vi "Format to Technique Parameters.vi"(8 "error in (no error)":errorcluster, 9 "Index":i32, 10 "Internal Technique Parameter":variant, 11 "Potentiostat Galvanostat in":refnum<class "Potentiostat Galvanostat.lvclass">) -> (0 "error out":errorcluster, 2 "Technique Parameters":T1[](array[typedef]) {"Parameter Type" items=["I32 (Long)", "BOOL (Boolean)", "SGL (Single Precision)"]}, 3 "Potentiostat Galvanostat out":refnum<class "Potentiostat Galvanostat.lvclass">)   [LabVIEW 2018, in "Potentiostat Galvanostat.lvclass"]
uses:
  Potentiostat Galvanostat.lvclass
  Controls/Technique Parameter.ctl
  Controls/Parameter Type.ctl
  Controls/Error Codes.ctl
  Potentiostat Galvanostat.lvclass/Potentiostat Galvanostat.ctl
  BL_GetErrorMsg.vi
  <vilib>/Utility/error.llb/Error Cluster From Error Code.vi
  <vilib>/Utility/Data Type/NI_Data Type.lvlib
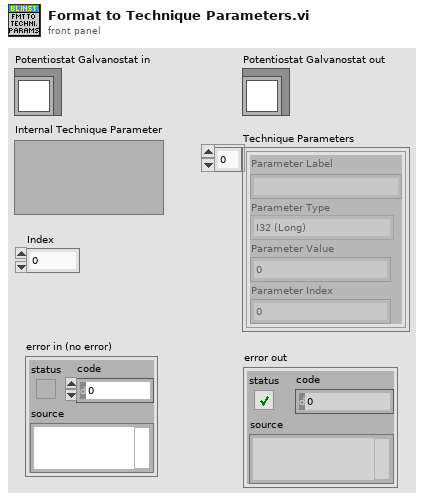
[diagram p1: front panel]
types:
  T1 = typedef "Potentiostat Galvanostat.lvclass/Technique Parameter.ctl" = cluster{"Parameter Label":string, "Parameter Type":T2, "Parameter Value":i32, "Parameter Index":i32}
  T2 = typedef "Potentiostat Galvanostat.lvclass/Parameter Type.ctl" = i32
  T3 = typedef "NI_Data Type.lvlib/Data Type.ctl" = enum8{"Invalid Type", "Void", "I8", "I16", "I32", "I64", "U8", "U16", "U32", "U64", "Single Float", "Double Float", "Extended Float", "Single Complex", "Double Complex", "Extended Complex", "Enum U8", "Enum U16", "Enum U32", "Enum U64", "Single Float With Unit", "Double Float With Unit", "Extended Float With Unit", "Single Complex with Unit", "Double Complex with Unit", "Extended Complex with Unit", "Boolean", "String", "Path", "Picture", "Tag", "Array", "Cluster", "Variant", "LV Variant", "Waveform", "Timestamp", "Digital Waveform", "Digital Data", "ExpressData", "Refnum", "External Data", "VI", "Poly VI", "LabVIEW Class Instance", "Fixed Point"}
  T4 = typedef "Potentiostat Galvanostat.lvclass/Error Codes.ctl" = i32
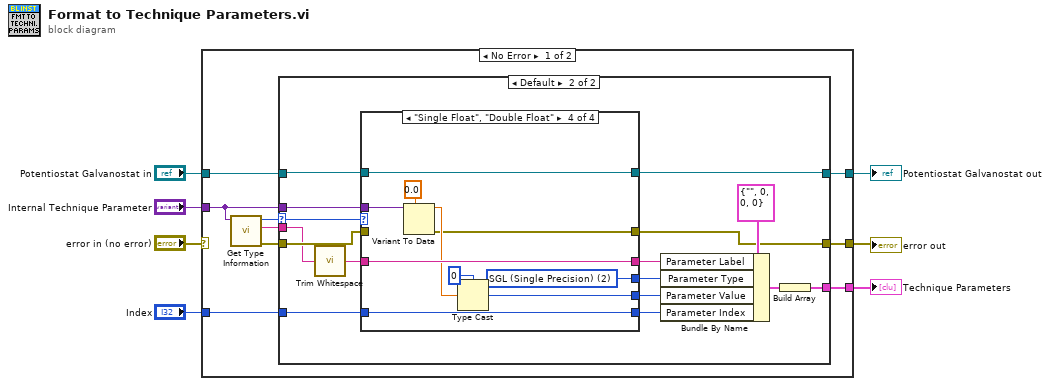
[diagram p0: block diagram]
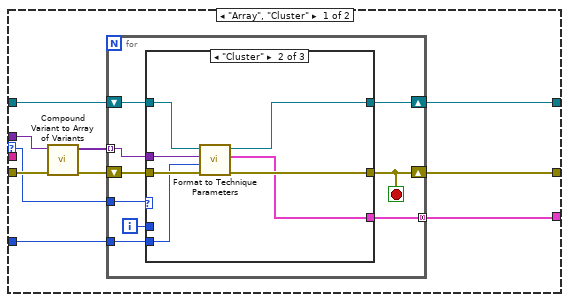
[diagram p2: hidden frame]
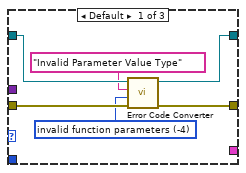
[diagram p3: hidden frame]
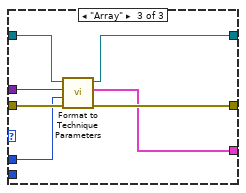
[diagram p4: hidden frame]
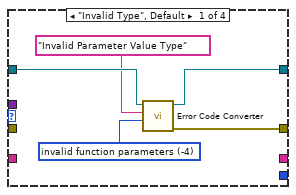
[diagram p5: hidden frame]
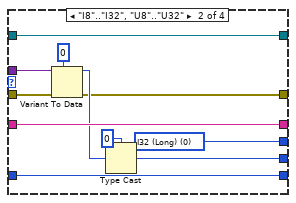
[diagram p6: hidden frame]
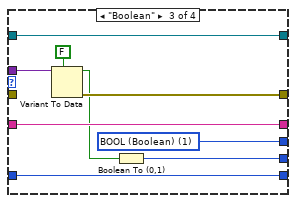
[diagram p7: hidden frame]
diagram:
  n1 = case shown="No Error" "error in (no error)" {
    selector: "error in (no error)" -> [_ w107]
    tunnel: "Internal Technique Parameter" -> [w15 _]
    tunnel: "Index" -> [w12 _]
    tunnel: "Potentiostat Galvanostat in" -> [w11 w108]
    tunnel: [w10 _] -> w4
    tunnel: [w9 w108] -> w3
    tunnel: [w8 w107] -> w2
    frame No Error {
      n2 = call <vilib>:"Get Type Information.vi"("Variant"=w15) -> ("error out"=w13:errorcluster, "Name"=w14:string, "Type"=w16:T3)  [unwired: 6 in, 2 out]
      n3 = case shown="Default" w16 {
        selector: w16 -> [w23 w62]
        tunnel: w15 -> [w26 w64]
        tunnel: w14 -> [_ w61]
        tunnel: w13 -> [w25 w63]
        tunnel: w12 -> [w20 w60]
        tunnel: w11 -> [w22 w65]
        tunnel: [w17 w59] -> w9
        tunnel: [w18 w56] -> w10
        tunnel: [w19 w58] -> w8
        frame "Array", "Cluster" {
          n4 = call "Compound Variant to Array of Variants.vi"("error in (no error)"=w25, "Array/Cluster Variant"=w26) -> ("error out"=w21:errorcluster, "[Variant]"=w24:variant[])  [unwired: 8 in]
          n5 = for {
            tunnel: w24 -> [w33] mode=indexing
            tunnel: w23 -> [w32]
            shift-right: [w29] -> w17
            shift-left: w22 -> [w34]
            shift-right: [w28] -> w19
            shift-left: w21 -> [w35]
            tunnel: w20 -> [w31]
            tunnel: [w30] -> w18 mode=concatenating
            i -> [w27]
            stop <- w28 stop-if-true
            n6 = case shown="\"Cluster\"" w32 {
              tunnel: w35 -> [w38 w48 w55]
              tunnel: w34 -> [w41 w47 w54]
              tunnel: w33 -> [_ w46 w53]
              tunnel: [w37 w45 w52] -> w28
              tunnel: w31 -> [_ w44 _]
              tunnel: [_ w43 w51] -> w30
              tunnel: [w39 w42 w50] -> w29
              tunnel: w27 -> [_ _ w49]
              frame Default {
                w36 = T4 -4 items=["No Error"=0, "no instrument connected"=-1, "connection in progress"=-2, "selected channel(s) unplugged"=-3, "invalid function parameters"=-4, "selected file does not exist"=-5, "function failed"=-6, "no channel selected"=-7, "invalid instrument configuration"=-8, "EC-Lab firmware loaded on the instrument"=-9, "library not correctly loaded in memory"=-10, "USB library not correctly loaded in memory"=-11, "function of the library already in progress"=-12, "selected channel(s) already used"=-13, "device not allowed"=-14, "Invalid update function parameters"=-15, "internal instrument communication failed"=-101, "too many data to transfer from the instrument (device error)"=-102, "selected channel(s) unplugged (device error)"=-103, "instrument response error"=-104, "invalid message size"=-105] ("Error Code")
                n7 = call "Error Code Converter.vi"("error in (no error)"=w38, "Error Code"=w36, "Additional Description"="Invalid Parameter Value Type", "Potentiostat Galvanostat in"=w41) -> ("error out"=w37:errorcluster, "Potentiostat Galvanostat out"=w39:refnum<class "Potentiostat Galvanostat.lvclass">)  [unwired: 6 in]
              }
              frame "Cluster" {
                n8 = call "Format to Technique Parameters.vi"("error in (no error)"=w48, "Index"=w44, "Internal Technique Parameter"=w46, "Potentiostat Galvanostat in"=w47) -> ("error out"=w45:errorcluster, "Technique Parameters"=w43:T1[], "Potentiostat Galvanostat out"=w42:refnum<class "Potentiostat Galvanostat.lvclass">)  [unwired: 5 in]
              }
              frame "Array" {
                n9 = call "Format to Technique Parameters.vi"("error in (no error)"=w55, "Index"=w49, "Internal Technique Parameter"=w53, "Potentiostat Galvanostat in"=w54) -> ("error out"=w52:errorcluster, "Technique Parameters"=w51:T1[], "Potentiostat Galvanostat out"=w50:refnum<class "Potentiostat Galvanostat.lvclass">)  [unwired: 5 in]
              }
            }
          }
        }
        frame Default {
          n10 = call <vilib>:"Trim Whitespace.vi"("string"=w61) -> ("trimmed string"=w71:string)  [unwired: 1 in]
          n11 = case shown="\"Single Float\", \"Double Float\"" w62 {
            tunnel: w64 -> [_ w87 w96 w106]
            tunnel: w65 -> [w76 w78 w90 w97]
            tunnel: [w75 w78 w90 w97] -> w59
            tunnel: [w74 w79 w91 w98] -> w58
            tunnel: w71 -> [_ w85 w94 w104]
            tunnel: w60 -> [_ w84 w93 w103]
            tunnel: [_ w85 w94 w104] -> w67
            tunnel: [_ w80 w92 w99] -> w68
            tunnel: [_ w83 w89 w102] -> w69
            tunnel: [_ w84 w93 w103] -> w70
            tunnel: w63 -> [_ w77 _ _]
            frame "Invalid Type", Default {
              w72 = T4 -4 items=["No Error"=0, "no instrument connected"=-1, "connection in progress"=-2, "selected channel(s) unplugged"=-3, "invalid function parameters"=-4, "selected file does not exist"=-5, "function failed"=-6, "no channel selected"=-7, "invalid instrument configuration"=-8, "EC-Lab firmware loaded on the instrument"=-9, "library not correctly loaded in memory"=-10, "USB library not correctly loaded in memory"=-11, "function of the library already in progress"=-12, "selected channel(s) already used"=-13, "device not allowed"=-14, "Invalid update function parameters"=-15, "internal instrument communication failed"=-101, "too many data to transfer from the instrument (device error)"=-102, "selected channel(s) unplugged (device error)"=-103, "instrument response error"=-104, "invalid message size"=-105] ("Error Code")
              n12 = call "Error Code Converter.vi"("Error Code"=w72, "Additional Description"="Invalid Parameter Value Type", "Potentiostat Galvanostat in"=w76) -> ("error out"=w74:errorcluster, "Potentiostat Galvanostat out"=w75:refnum<class "Potentiostat Galvanostat.lvclass">)  [unwired: 7 in]
            }
            frame "I8".."I32", "U8".."U32" {
              w80 = T2 0 items=["I32 (Long)", "BOOL (Boolean)", "SGL (Single Precision)"] ("Parameter Type")
              n13 = Variant To Data(error in=w77, type=0, Variant=w87) -> (data=w81:i32, error out=w79:errorcluster)
              n14 = Type Cast(type=0, x=w81) -> (*(type *) &x=w83:i32)
            }
            frame "Boolean" {
              w92 = T2 1 items=["I32 (Long)", "BOOL (Boolean)", "SGL (Single Precision)"] ("Parameter Type")
              n15 = Variant To Data(type=FALSE, Variant=w96) -> (data=w88:bool, error out=w91:errorcluster)  [unwired: 1 in]
              n16 = Boolean To (0,1)(Boolean=w88) -> (0, 1=w89:i16)
            }
            frame "Single Float", "Double Float" {
              w99 = T2 2 items=["I32 (Long)", "BOOL (Boolean)", "SGL (Single Precision)"] ("Parameter Type")
              n17 = Variant To Data(type=sgl 0.0 ("Numeric"), Variant=w106) -> (data=w100:sgl, error out=w98:errorcluster)  [unwired: 1 in]
              n18 = Type Cast(type=0, x=w100) -> (*(type *) &x=w102:i32)
            }
          }
          n19 = Bundle By Name(cluster=T1 {"Parameter Label"="", "Parameter Type"=0, "Parameter Value"=0, "Parameter Index"=0} ("Technique Parameter"), "Parameter Label"=w67, "Parameter Type"=w68, "Parameter Value"=w69, "Parameter Index"=w70) -> (w57:T1)
          n20 = Build Array(w57) -> (w56:T1[])
        }
      }
    }
    frame Error {
    }
  }
  "Technique Parameters" <- w4
  "Potentiostat Galvanostat out" <- w3
  "error out" <- w2
